vi "DisplayPanel.vi"() -> ()   [LabVIEW 2015]
uses:
  MvLVLib/VIs/CreateU3VHandle.vi
  MvLVLib/VIs/CreateGigEHandle.vi
  MvLVLib/MvCameraControl.lvlib
panel:
  out "Image":T1(plugin-control)
  out "U3VDeviceArray":T2(array[cluster])
  out "GigEDeviceArray":T3(array[cluster])
  in  "pConvertInfo In":T4
  out "PixelFormat":u32
  out "handle out":u64
  in  "handle":u64
  out "PayloadSize":u32
  out "pFrameInfoEx out":T5
  out "nHeight":u32
  out "nWidth":u32
  out "Acquisision Flag":bool
  in  "Trigger Mode":bool
  in  "Continuous":bool
  out "打开标志":bool
  in  "stop":bool
  in  "Trigger Once":bool
  in  "Stop":bool
  in  "Start":bool
  in  "Open Device":bool
  in  "Close Device":bool
  in  "error in (no error) 2":errorcluster caption="错误输入（无错误）"
  in  "Refresh Devices":bool
  in  "Device List":u16(ring) items=["[U3V] _322_sfs_含    22& MV-CS060-10UC-PRO(L25341278)"]
  # "Initialize"
  # "Acquisition"
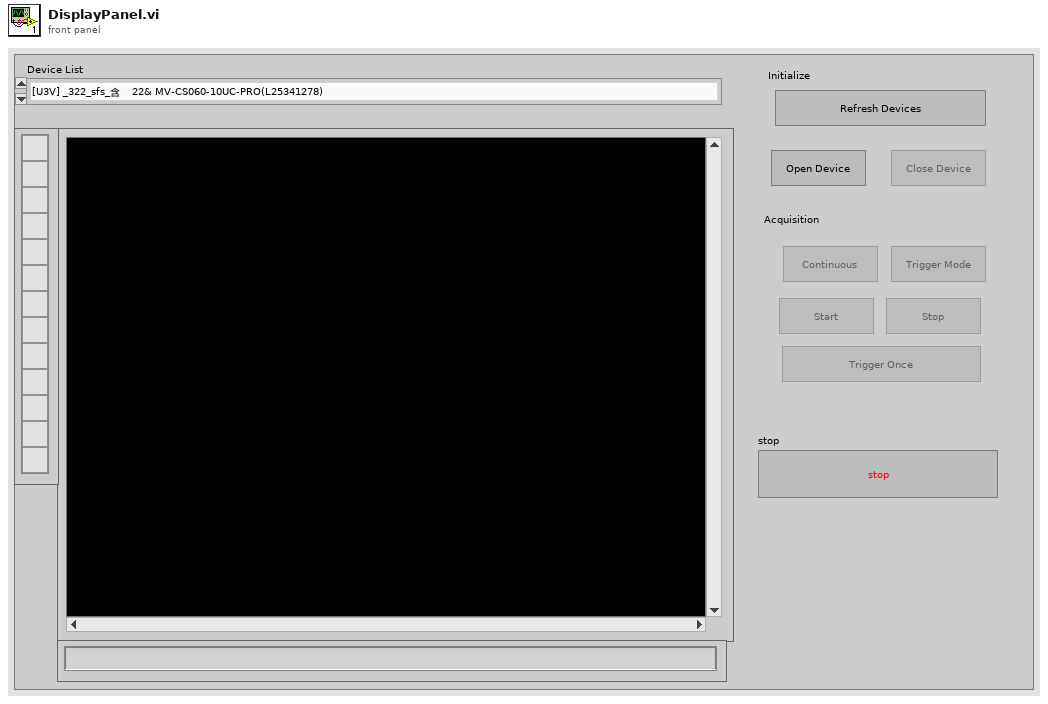
[diagram p1: front panel]
types:
  T1 = typedef "IMAQ Image.ctl" = refnum<image>
  T2 = cluster{"nMajorVer":u16, "nMinorVer":u16, "nMacAddrHigh":u32, "nMacAddrLow":u32, "nTLayerType":u32, "nReserved0":u32, "nReserved1":u32, "nReserved2":u32, "nReserved3":u32, "CrtlInEndPoint":u8, "CrtlOutEndPoint":u8, "StreamEndPoint":u8, "EventEndPoint":u8, "idVendor":u16, "idProduct":u16, "nDeviceNumber":u32, "chDeviceGUID":string, "chVendorName":string, "chModelName":string, "chFamilyName":string, "chDeviceVersion":string, "chManufacturerName":string, "chSerialNumber":string, "chUserDefinedName":string, "nbcdUSB":u32, "nDeviceAddress":u32, "nRes0":u32, "nRes1":u32, "nResAlign":u32}[]
  T3 = cluster{"nMajorVer":u16, "nMinorVer":u16, "nMacAddrHigh":u32, "nMacAddrLow":u32, "nTLayerType":u32, "nReserved0":u32, "nReserved1":u32, "nReserved2":u32, "nReserved3":u32, "nIpCfgOption":u32, "nIpCfgCurrent":u32, "nCurrentIp":u32, "nCurrentSubNetMask":u32, "nDefaultGateWay":u32, "chManualfacturerName":string, "chModelName":string, "chDeviceVersion":string, "chManufacturerSpecificInfo":string, "chSerialNumber":string, "chUserDefinedName":string, "nNetExport":u32, "nRes0":u32, "nRes1":u32, "nRes2":u32, "nRes3":u32}[]
  T4 = cluster{"nWidth":u16, "nHeight":u16, "enSrcPixelType":u32, "nSrcDataLen":u32, "enDstPixelType":u32, "nDstLen":u32, "nDstBufferSize":u32, "nRes0":u32, "nRes1":u32, "nRes2":u32, "nRes3":u32}
  T5 = cluster{"nWidth":u16, "nHeight":u16, "enPixelType":i32, "nFrameNum":u32, "nDevTimeStampHigh":u32, "nDevTimeStampLow":u32, "nReserved0":u32, "nHostTimeStamp":i64, "nFrameLen":u32, "nSecondCount]":u32, "nCycleCount":u32, "nCycleOffset":u32, "fGain":u32, "fExposureTime":u32, "nAverageBrightness":u32, "nRed":u32, "nGreen":u32, "nBlue":u32, "nFrameCounter":u32, "nTriggerIndex":u32, "nInput":u32, "nOutput":u32, "nOffsetX":u32, "nOffsetY":u32, "nReserved[0]":u32, "nReserved[1]":u32, "nReserved[2]":u32, "nReserved[3]":u32, "nReserved[4]":u32, "nReserved[5]":u32, "nReserved[6]":u32, "nReserved[7]":u32, "nReserved[8]":u32, "nReserved[9]":u32, "nReserved[10]":u32, "nReserved[11]":u32, "nReserved[12]":u32, "nReserved[13]":u32, "nReserved[14] 10":u32, "nReserved[15] 11":u32, "nReserved[16] 12":u32, "nReserved[17] 13":u32, "nReserved[18] 14":u32, "nReserved[19] 15":u32, "nReserved[20] 16":u32, "nReserved[21] 17":u32, "nReserved[22] 18":u32, "nReserved[23] 19":u32, "nReserved[24] 20":u32, "nReserved[25] 21":u32, "nReserved[26] 22":u32, "nReserved[27] 23":u32, "nReserved[28] 24":u32, "nReserved[29] 25":u32, "nReserved[30] 26":u32, "nReserved[31] 27":u32, "nReserved[32] 28":u32, "nReserved[33] 29":u32, "nReserved[34] 30":u32, "nReserved[35] 31":u32, "nReserved[36] 32":u32, "nReserved[37] 33":u32, "nReserved[38] 34":u32, "nReserved[39] 35":u32, "nReserved[40] 36":u32}
  T6 = enum8{"Enabled", "Disabled", "Disabled and Grayed Out"}
  T7 = cluster{"nCurValue":u32, "nMax":u32, "nMin":u32, "nInc":u32, "nReserved[0]":u32, "nReserved[1]":u32, "nReserved[2]":u32, "nReserved[3]":u32}
  T8 = cluster{"nCurValue":u32, "nSupportedNum":u32, "nSupportValue[0]":u32, "nSupportValue[1]":u32, "nSupportValue[2]":u32, "nSupportValue[3]":u32, "nSupportValue[4]":u32, "nSupportValue[5]":u32, "nSupportValue[6]":u32, "nSupportValue[7]":u32, "nSupportValue[8]":u32, "nSupportValue[9]":u32, "nSupportValue[10]":u32, "nSupportValue[11]":u32, "nSupportValue[12]":u32, "nSupportValue[13]":u32, "nSupportValue[14]":u32, "nSupportValue[15]":u32, "nSupportValue[16]":u32, "nSupportValue[17]":u32, "nSupportValue[18]":u32, "nSupportValue[19]":u32, "nSupportValue[20]":u32, "nSupportValue[21]":u32, "nSupportValue[22]":u32, "nSupportValue[23]":u32, "nSupportValue[24]":u32, "nSupportValue[25]":u32, "nSupportValue[26]":u32, "nSupportValue[27]":u32, "nSupportValue[28]":u32, "nSupportValue[29]":u32, "nSupportValue[30]":u32, "nSupportValue[31]":u32, "nSupportValue[32]":u32, "nSupportValue[33]":u32, "nSupportValue[34]":u32, "nSupportValue[35]":u32, "nSupportValue[36]":u32, "nSupportValue[37]":u32, "nSupportValue[38]":u32, "nSupportValue[39]":u32, "nSupportValue[40]":u32, "nSupportValue[41]":u32, "nSupportValue[42]":u32, "nSupportValue[43]":u32, "nSupportValue[44]":u32, "nSupportValue[45]":u32, "nSupportValue[46]":u32, "nSupportValue[47]":u32, "nSupportValue[48]":u32, "nSupportValue[49]":u32, "nSupportValue[50]":u32, "nSupportValue[51]":u32, "nSupportValue[52]":u32, "nSupportValue[53]":u32, "nSupportValue[54]":u32, "nSupportValue[55]":u32, "nSupportValue[56]":u32, "nSupportValue[57]":u32, "nSupportValue[58]":u32, "nSupportValue[59]":u32, "nSupportValue[60]":u32, "nSupportValue[61]":u32, "nSupportValue[62]":u32, "nSupportValue[63]":u32, "nReserved[0]":u32, "nReserved[1]":u32, "nReserved[2]":u32, "nReserved[3]":u32}
  T9 = typedef "Image Type" = u32
  T10 = cluster{"nMajorVer":u16, "nMinorVer":u16, "nMacAddrHigh":u32, "nMacAddrLow":u32, "nTLayerType":u32, "nReserved0":u32, "nReserved1":u32, "nReserved2":u32, "nReserved3":u32, "CrtlInEndPoint":u8, "CrtlOutEndPoint":u8, "StreamEndPoint":u8, "EventEndPoint":u8, "idVendor":u16, "idProduct":u16, "nDeviceNumber":u32, "chDeviceGUID":string, "chVendorName":string, "chModelName":string, "chFamilyName":string, "chDeviceVersion":string, "chManufacturerName":string, "chSerialNumber":string, "chUserDefinedName":string, "nbcdUSB":u32, "nDeviceAddress":u32, "nRes0":u32, "nRes1":u32, "nResAlign":u32}
  T11 = cluster{"nMajorVer":u16, "nMinorVer":u16, "nMacAddrHigh":u32, "nMacAddrLow":u32, "nTLayerType":u32, "nReserved0":u32, "nReserved1":u32, "nReserved2":u32, "nReserved3":u32, "nIpCfgOption":u32, "nIpCfgCurrent":u32, "nCurrentIp":u32, "nCurrentSubNetMask":u32, "nDefaultGateWay":u32, "chManualfacturerName":string, "chModelName":string, "chDeviceVersion":string, "chManufacturerSpecificInfo":string, "chSerialNumber":string, "chUserDefinedName":string, "nNetExport":u32, "nRes0":u32, "nRes1":u32, "nRes2":u32, "nRes3":u32}
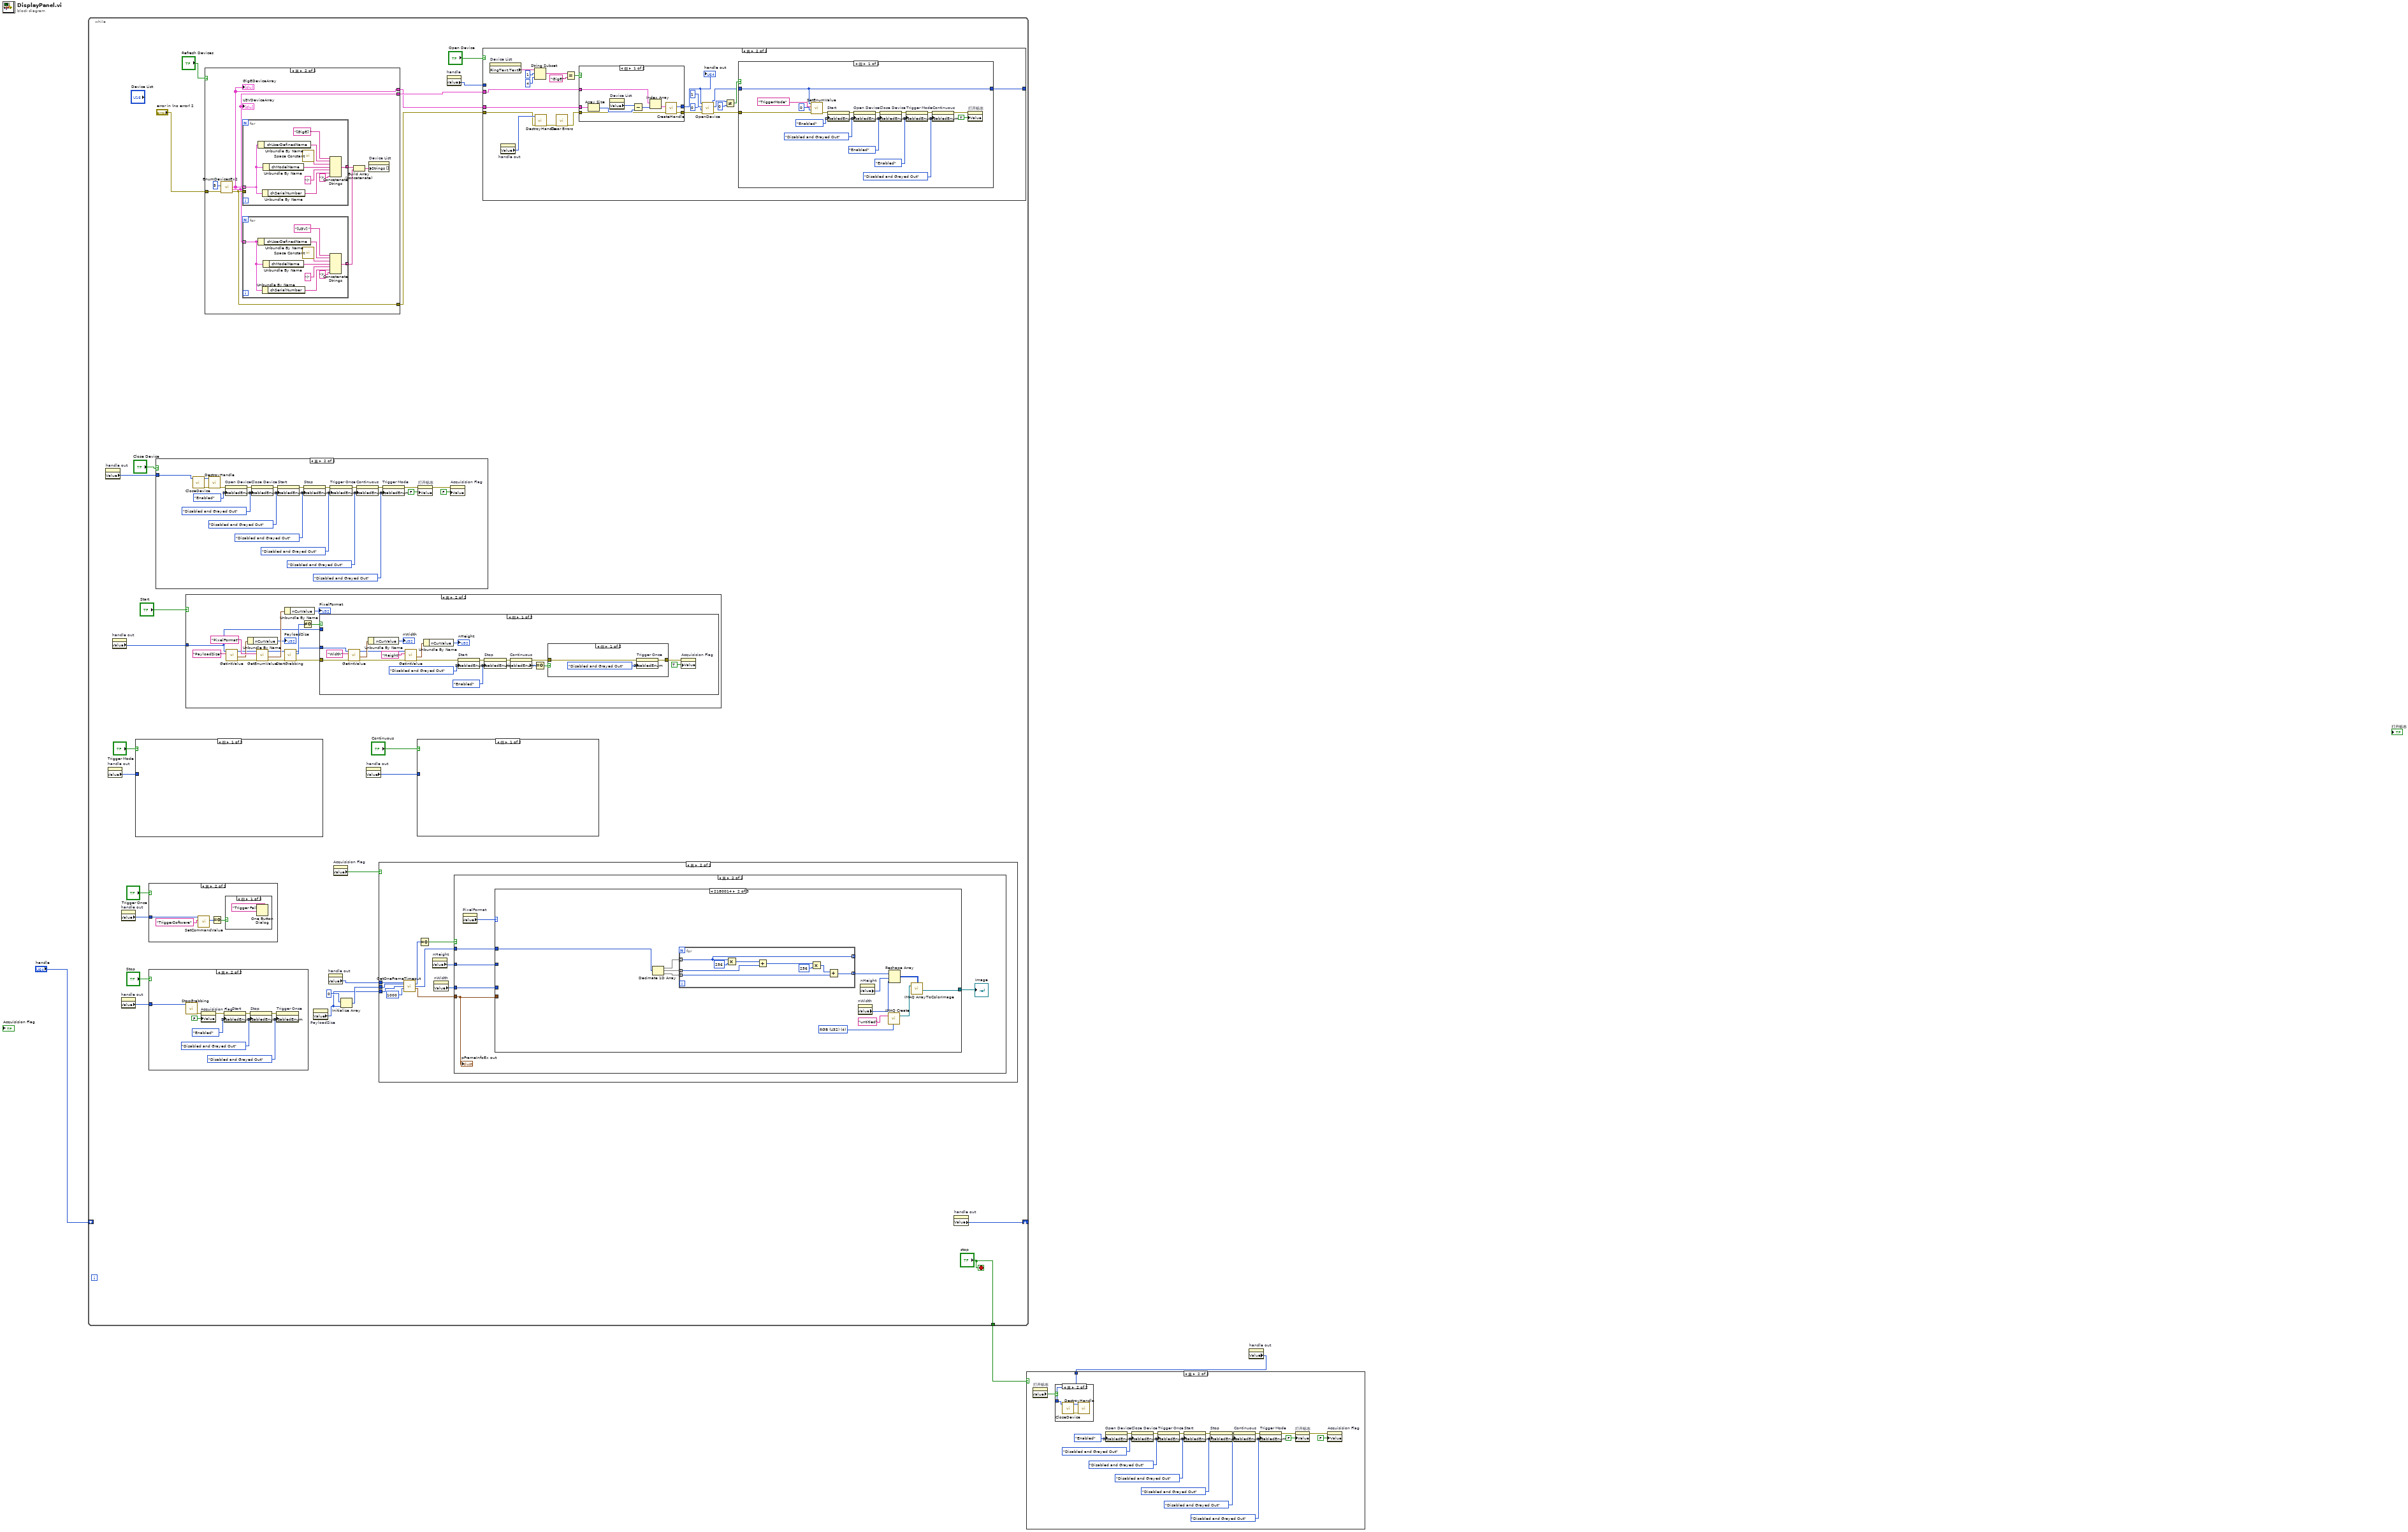
[diagram p0: block diagram]
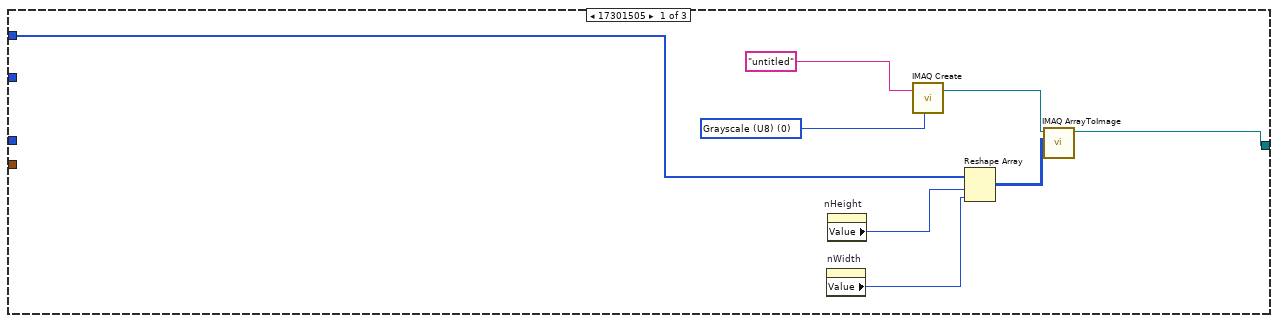
[diagram p6: hidden frame]
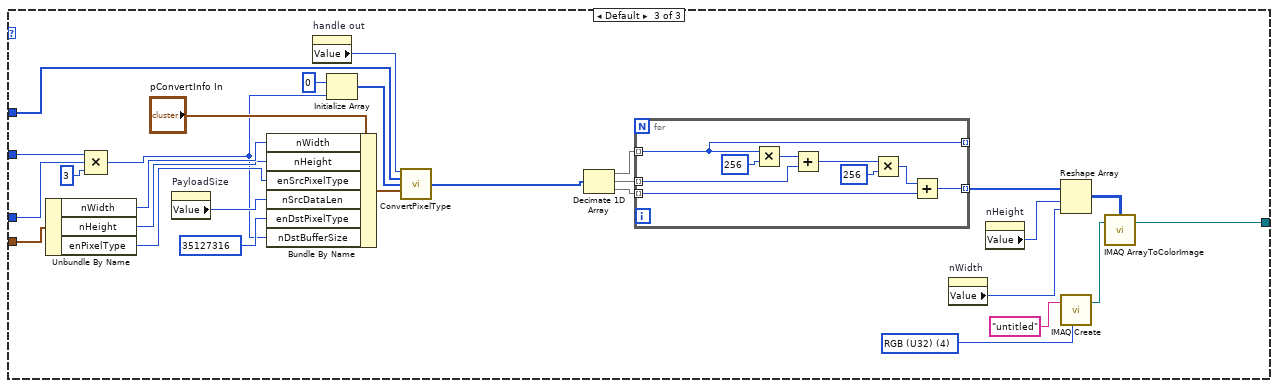
[diagram p7: hidden frame]
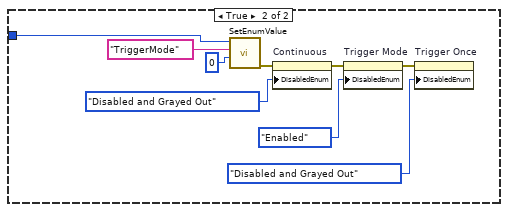
[diagram p9: hidden frame]
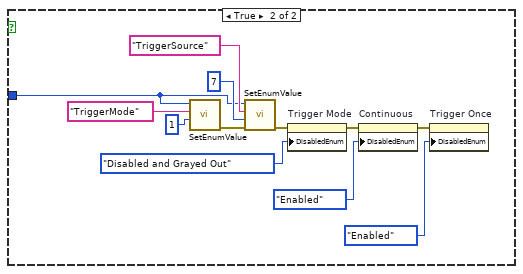
[diagram p10: hidden frame]
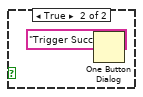
[diagram p12: hidden frame]
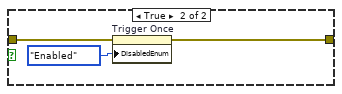
[diagram p14: hidden frame]
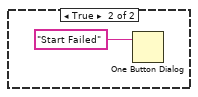
[diagram p15: hidden frame]
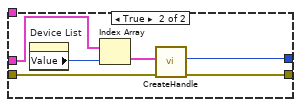
[diagram p18: hidden frame]
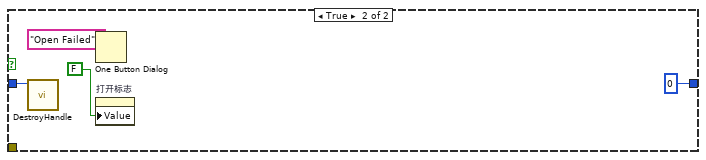
[diagram p19: hidden frame]
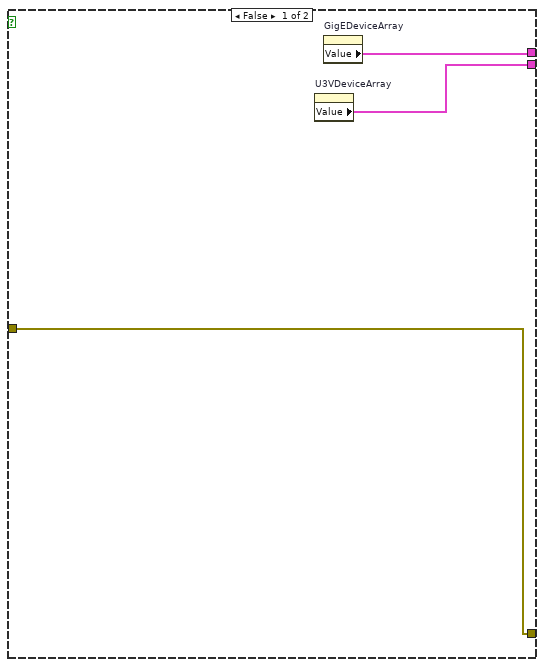
[diagram p20: hidden frame]
diagram:
  n1 = while {
    tunnel: ["stop"] -> w3
    shift-right: [w17] -> _
    shift-left: "handle" -> [_]
    stop <- "stop" stop-if-true
    n2 = property on="handle out" class="DigNum (严格)"() -> ("Value"=w15:u64)  [unwired: 2 in, 2 out]
    n3 = property on="handle out" class="DigNum (严格)"() -> ("Value"=w10:u64)  [unwired: 2 in, 2 out]
    n4 = property on="handle out" class="DigNum (严格)"() -> ("Value"=w11:u64)  [unwired: 2 in, 2 out]
    n5 = property on="handle out" class="DigNum (严格)"() -> ("Value"=w14:u64)  [unwired: 2 in, 2 out]
    n6 = property on="handle out" class="DigNum (严格)"() -> ("Value"=w13:u64)  [unwired: 2 in, 2 out]
    n7 = case shown="假" "Trigger Mode" {
      tunnel: w10 -> [_ w130]
      frame False {
      }
      frame True {
        n8 = call "SetEnumValue.vi"("nValue"=u32 1, "strKey"="TriggerMode", "handle"=w130) -> ("error out"=w136:errorcluster)  [unwired: 6 in, 2 out]
        n9 = call "SetEnumValue.vi"("error in (no error)"=w136, "nValue"=u32 7, "strKey"="TriggerSource", "handle"=w130) -> ("error out"=w135:errorcluster)  [unwired: 5 in, 2 out]
        n10 = property on="Trigger Mode" class="Bool"(error in=w135, "DisabledEnum"=T6."Disabled and Grayed Out" ("禁用")) -> (error out=w134:errorcluster)  [unwired: 1 in, 1 out]
        n11 = property on="Continuous" class="Bool"(error in=w134, "DisabledEnum"=T6."Enabled" ("禁用")) -> (error out=w132:errorcluster)  [unwired: 1 in, 1 out]
        n12 = property on="Trigger Once" class="Bool"(error in=w132, "DisabledEnum"=T6."Enabled" ("禁用")) -> ()  [unwired: 1 in, 2 out]
      }
    }
    n13 = case shown="真" "Trigger Once" {
      tunnel: w14 -> [_ w145]
      frame False {
      }
      frame True {
        n14 = call "SetCommandValue.vi"("strValue"="TriggerSoftware", "handle"=w145) -> ("function return"=w143:i32)  [unwired: 7 in, 2 out]
        n15 = Equal To 0?(x=w143) -> (x = 0?=w142:bool)
        n16 = case shown="假" w142 {
          frame False {
            n17 = One Button Dialog(message="Trigger Failed") -> ()  [unwired: 1 in, 1 out]
          }
          frame True {
            n18 = One Button Dialog(message="Trigger Success") -> ()  [unwired: 1 in, 1 out]
          }
        }
      }
    }
    n19 = case shown="真" "Stop" {
      tunnel: w13 -> [_ w120]
      frame False {
      }
      frame True {
        n20 = call "StopGrabbing.vi"("handle"=w120) -> ("error out"=w119:errorcluster)  [unwired: 8 in, 2 out]
        n21 = property on="Acquisision Flag" class="Bool (严格)"(error in=w119, "Value"=FALSE ("采集标志")) -> (error out=w114:errorcluster)  [unwired: 1 in, 1 out]
        n22 = property on="Start" class="Bool"(error in=w114, "DisabledEnum"=T6."Enabled" ("禁用")) -> (error out=w113:errorcluster)  [unwired: 1 in, 1 out]
        n23 = property on="Stop" class="Bool"(error in=w113, "DisabledEnum"=T6."Disabled and Grayed Out" ("禁用")) -> (error out=w112:errorcluster)  [unwired: 1 in, 1 out]
        n24 = property on="Trigger Once" class="Bool"(error in=w112, "DisabledEnum"=T6."Disabled and Grayed Out" ("禁用")) -> ()  [unwired: 1 in, 2 out]
      }
    }
    n25 = case shown="真" "Close Device" {
      tunnel: w15 -> [_ w191]
      frame False {
      }
      frame True {
        n26 = call "CloseDevice.vi"("handle"=w191) -> ("error out"=w193:errorcluster, "handle out"=w190:u64)  [unwired: 8 in, 1 out]
        n27 = call "DestroyHandle.vi"("error in (no error)"=w193, "handle"=w190) -> ("error out"=w192:errorcluster)  [unwired: 8 in, 1 out]
        n28 = property on="Open Device" class="Bool"(error in=w192, "DisabledEnum"=T6."Enabled" ("禁用")) -> (error out=w206:errorcluster)  [unwired: 1 in, 1 out]
        n29 = property on="Close Device" class="Bool"(error in=w206, "DisabledEnum"=T6."Disabled and Grayed Out" ("禁用")) -> (error out=w205:errorcluster)  [unwired: 1 in, 1 out]
        n30 = property on="Start" class="Bool"(error in=w205, "DisabledEnum"=T6."Disabled and Grayed Out" ("禁用")) -> (error out=w204:errorcluster)  [unwired: 1 in, 1 out]
        n31 = property on="Stop" class="Bool"(error in=w204, "DisabledEnum"=T6."Disabled and Grayed Out" ("禁用")) -> (error out=w203:errorcluster)  [unwired: 1 in, 1 out]
        n32 = property on="Trigger Once" class="Bool"(error in=w203, "DisabledEnum"=T6."Disabled and Grayed Out" ("禁用")) -> (error out=w200:errorcluster)  [unwired: 1 in, 1 out]
        n33 = property on="Continuous" class="Bool"(error in=w200, "DisabledEnum"=T6."Disabled and Grayed Out" ("禁用")) -> (error out=w198:errorcluster)  [unwired: 1 in, 1 out]
        n34 = property on="Trigger Mode" class="Bool"(error in=w198, "DisabledEnum"=T6."Disabled and Grayed Out" ("禁用")) -> (error out=w197:errorcluster)  [unwired: 1 in, 1 out]
        n35 = property on="打开标志" class="Bool (严格)"(error in=w197, "Value"=FALSE ("打开标志")) -> (error out=w195:errorcluster)  [unwired: 1 in, 1 out]
        n36 = property on="Acquisision Flag" class="Bool (严格)"(error in=w195, "Value"=FALSE ("采集标志")) -> ()  [unwired: 1 in, 2 out]
      }
    }
    n37 = case shown="真" "Start" {
      tunnel: w11 -> [_ w152]
      frame False {
      }
      frame True {
        n38 = call "GetIntValue.vi"("strKey"="PayloadSize", "handle"=w152) -> ("error out"=w158:errorcluster, "pIntValue out"=w154:T7, "handle out"=w150:u64)  [unwired: 6 in, 1 out]
        n39 = Unbundle By Name(w154) -> ("nCurValue"=→"PayloadSize":u32)
        n40 = call "GetEnumValue.vi"("error in (no error)"=w158, "strKey"="PixelFormat", "handle"=w150) -> ("error out"=w157:errorcluster, "pEnumValue out"=w159:T8, "handle out"=w149:u64)  [unwired: 5 in, 1 out]
        n41 = Unbundle By Name(w159) -> ("nCurValue"=→"PixelFormat":u32)
        n42 = call "StartGrabbing.vi"("error in (no error)"=w157, "handle"=w149) -> ("error out"=w156:errorcluster, "function return"=w162:i32, "handle out"=w148:u64)  [unwired: 7 in]
        n43 = Not Equal To 0?(x=w162) -> (x != 0?=w161:bool)
        n44 = case shown="假" w161 {
          tunnel: w152 -> [_ _]
          tunnel: w156 -> [w165 _]
          tunnel: w148 -> [w164 _]
          frame False {
            n45 = call "GetIntValue.vi"("error in (no error)"=w165, "strKey"="Width", "handle"=w164) -> ("error out"=w172:errorcluster, "pIntValue out"=w166:T7, "handle out"=w163:u64)  [unwired: 5 in, 1 out]
            n46 = Unbundle By Name(w166) -> ("nCurValue"=→"nWidth":u32)
            n47 = call "GetIntValue.vi"("error in (no error)"=w172, "strKey"="Height", "handle"=w163) -> ("error out"=w171:errorcluster, "pIntValue out"=w169:T7)  [unwired: 5 in, 2 out]
            n48 = Unbundle By Name(w169) -> ("nCurValue"=→"nHeight":u32)
            n49 = property on="Start" class="Bool"(error in=w171, "DisabledEnum"=T6."Disabled and Grayed Out" ("禁用")) -> (error out=w181:errorcluster)  [unwired: 1 in, 1 out]
            n50 = property on="Stop" class="Bool"(error in=w181, "DisabledEnum"=T6."Enabled" ("禁用")) -> (error out=w167:errorcluster)  [unwired: 1 in, 1 out]
            n51 = property on="Continuous" class="Bool"(error in=w167) -> (error out=w177:errorcluster, "DisabledEnum"=w178:T6)  [unwired: 1 in, 1 out]
            n52 = Equal To 0?(x=w178) -> (x = 0?=w179:bool)
            n53 = case shown="假" w179 {
              tunnel: w177 -> [w184 w187]
              tunnel: [w183 w186] -> w176
              frame False {
                n54 = property on="Trigger Once" class="Bool"(error in=w184, "DisabledEnum"=T6."Disabled and Grayed Out" ("禁用")) -> (error out=w183:errorcluster)  [unwired: 1 in, 1 out]
              }
              frame True {
                n55 = property on="Trigger Once" class="Bool"(error in=w187, "DisabledEnum"=T6."Enabled" ("禁用")) -> (error out=w186:errorcluster)  [unwired: 1 in, 1 out]
              }
            }
            n56 = property on="Acquisision Flag" class="Bool (严格)"(error in=w176, "Value"=TRUE ("采集标志")) -> ()  [unwired: 1 in, 2 out]
          }
          frame True {
            n57 = One Button Dialog(message="Start Failed") -> ()  [unwired: 1 in, 1 out]
          }
        }
      }
    }
    n58 = case shown="真" "Refresh Devices" {
      tunnel: [w271 w279] -> w19
      tunnel: "error in (no error) 2" -> [w271 w278]
      tunnel: [w269 w273] -> w5
      tunnel: [w270 w274] -> w4
      frame False {
        n59 = property on="U3VDeviceArray" class="Arr (严格)"() -> ("Value"=w269:T2)  [unwired: 2 in, 2 out]
        n60 = property on="GigEDeviceArray" class="Arr (严格)"() -> ("Value"=w270:T3)  [unwired: 2 in, 2 out]
      }
      frame True {
        n61 = call "EnumDevicesEx2.vi"("nLayerType"=5, "error in (no error)"=w278) -> ("GigEDeviceArray"=w274:T3, "U3VDeviceArray"=w273:T2, "error out"=w279:errorcluster)  [unwired: 9 in, 2 out]
        "GigEDeviceArray" <- w274
        "U3VDeviceArray" <- w273
        n62 = for {
          tunnel: w279 -> [_]
          tunnel: w274 -> [w291] mode=indexing
          tunnel: [w290] -> w277 mode=indexing
          n63 = Unbundle By Name(w291) -> ("chUserDefinedName"=w294:string)
          n64 = Unbundle By Name(w291) -> ("chSerialNumber"=w292:string)
          n65 = Unbundle By Name(w291) -> ("chModelName"=w293:string)
          n66 = call <vilib>:"Space Constant.vi"() -> ("String"=w297:string)
          n67 = Concatenate Strings("[GigE] " ("字符串"), w294, w297, w293, "(" ("字符串"), w292, ")" ("字符串")) -> (w290:string)
        }
        n68 = for {
          tunnel: w273 -> [w284] mode=indexing
          tunnel: [w281] -> w276 mode=indexing
          n69 = Unbundle By Name(w284) -> ("chUserDefinedName"=w288:string)
          n70 = Unbundle By Name(w284) -> ("chSerialNumber"=w283:string)
          n71 = Unbundle By Name(w284) -> ("chModelName"=w286:string)
          n72 = call <vilib>:"Space Constant.vi"() -> ("String"=w287:string)
          n73 = Concatenate Strings("[U3V] " ("字符串"), w288, w287, w286, "(" ("字符串"), w283, ")" ("字符串")) -> (w281:string)
        }
        n74 = Build Array (concatenate)(w277, w276) -> (w275:string[])
        n75 = property on="Device List" class="Ring (严格)"("Strings []"=w275) -> ()  [unwired: 2 in, 2 out]
      }
    }
    n76 = property on="PayloadSize" class="DigNum (严格)"() -> ("Value"=w6:u32)  [unwired: 2 in, 2 out]
    n77 = property on="handle out" class="DigNum (严格)"() -> ("Value"=w12:u64)  [unwired: 2 in, 2 out]
    n78 = property on="Acquisision Flag" class="Bool (严格)"() -> ("Value"=w21:bool)  [unwired: 2 in, 2 out]
    n79 = Initialize Array(u8 0 ("元素"), w6) -> (w7:u8[])
    n80 = property on="handle out" class="DigNum (严格)"() -> ("Value"=w9:u64)  [unwired: 2 in, 2 out]
    n81 = case shown="真" w21 {
      tunnel: w12 -> [_ w35]
      tunnel: w7 -> [_ w34]
      tunnel: w6 -> [_ w33]
      frame False {
      }
      frame True {
        n82 = call "GetOneFrameTimeout.vi"("handle"=w35, "pData"=w34, "nDataSize"=w33, "nMsec"=1000) -> ("function return"=w32:i32, "pData Out"=w31:u8[], "pFrameInfoEx out"=w30:T5)  [unwired: 7 in, 2 out]
        n83 = Equal To 0?(x=w32) -> (x = 0?=w39:bool)
        n84 = property on="nHeight" class="DigNum (严格)"() -> ("Value"=w37:u32)  [unwired: 2 in, 2 out]
        n85 = property on="nWidth" class="DigNum (严格)"() -> ("Value"=w38:u32)  [unwired: 2 in, 2 out]
        n86 = case shown="真" w39 {
          tunnel: w31 -> [_ w45]
          tunnel: w38 -> [_ w43]
          tunnel: w37 -> [_ w44]
          tunnel: w30 -> [_ w41]
          frame False {
          }
          frame True {
            n87 = property on="PixelFormat" class="DigNum (严格)"() -> ("Value"=w42:u32)  [unwired: 2 in, 2 out]
            n88 = case shown="2180014" w42 {
              tunnel: w45 -> [w46 w57 w99]
              tunnel: w44 -> [_ _ w96]
              tunnel: w43 -> [_ _ w95]
              tunnel: w41 -> [_ _ w87]
              tunnel: [w47 w56 w75] -> w40
              frame 17301505 {
                w53 = T9 0 items=["Grayscale (U8)", "Grayscale (I16)", "Grayscale (SGL)", "Complex (CSG)", "RGB (U32)", "HSL (U32)", "RGB (U64)", "Grayscale (U16)"] ("Image Type")
                n89 = property on="nWidth" class="DigNum (严格)"() -> ("Value"=w48:u32)  [unwired: 2 in, 2 out]
                n90 = property on="nHeight" class="DigNum (严格)"() -> ("Value"=w49:u32)  [unwired: 2 in, 2 out]
                n91 = call "IMAQ Create"("Image Name"="untitled", "Image Type"=w53) -> ("New Image"=w51:T1)  [unwired: 3 in, 1 out]
                n92 = Reshape Array(w46, w49, w48) -> (w50:u8[][])
                n93 = call "IMAQ ArrayToImage"("Image Pixels (U8)"=w50, "Image"=w51) -> ("Image Out"=w47:T1)  [unwired: 8 in, 1 out]
              }
              frame 35127316 {
                w65 = T9 4 items=["Grayscale (U8)", "Grayscale (I16)", "Grayscale (SGL)", "Complex (CSG)", "RGB (U32)", "HSL (U32)", "RGB (U64)", "Grayscale (U16)"] ("Image Type")
                n94 = Decimate 1D Array(w57) -> (w58:u8[], w59:u8[], w60:u8[])
                n95 = for {
                  tunnel: w58 -> [w66] mode=indexing
                  tunnel: w59 -> [w72] mode=indexing
                  tunnel: w60 -> [w68] mode=indexing
                  tunnel: [w67] -> w61 mode=indexing
                  tunnel: [w66] -> _ mode=indexing
                  n96 = Multiply(x=w66, y=256) -> (x*y=w73:i32)
                  n97 = Add(x=w73, y=w72) -> (x+y=w71:i32)
                  n98 = Multiply(x=w71, y=256) -> (x*y=w69:i32)
                  n99 = Add(x=w69, y=w68) -> (x+y=w67:i32)
                }
                n100 = property on="nWidth" class="DigNum (严格)"() -> ("Value"=w54:u32)  [unwired: 2 in, 2 out]
                n101 = property on="nHeight" class="DigNum (严格)"() -> ("Value"=w55:u32)  [unwired: 2 in, 2 out]
                n102 = call "IMAQ Create"("Image Name"="untitled", "Image Type"=w65) -> ("New Image"=w63:T1)  [unwired: 3 in, 1 out]
                n103 = Reshape Array(w61, w55, w54) -> (w62:i32[][])
                n104 = call "IMAQ ArrayToColorImage"("Image Pixels (U32)"=w62, "Image"=w63) -> ("Image Out"=w56:T1)  [unwired: 3 in, 1 out]
              }
              frame Default {
                w86 = T9 4 items=["Grayscale (U8)", "Grayscale (I16)", "Grayscale (SGL)", "Complex (CSG)", "RGB (U32)", "HSL (U32)", "RGB (U64)", "Grayscale (U16)"] ("Image Type")
                n105 = Unbundle By Name(w87) -> ("nWidth"=w94:u16, "nHeight"=w93:u16, "enPixelType"=w92:i32)
                n106 = Compound Arithmetic op=MULTIPLY(w96, w95, u32 3 ("值")) -> (w89:u32)
                n107 = property on="PayloadSize" class="DigNum (严格)"() -> ("Value"=w91:u32)  [unwired: 2 in, 2 out]
                n108 = Bundle By Name(cluster="pConvertInfo In", "nWidth"=w94, "nHeight"=w93, "enSrcPixelType"=w92, "nSrcDataLen"=w91, "enDstPixelType"=u32 35127316, "nDstBufferSize"=w89) -> (w88:T4)
                n109 = property on="handle out" class="DigNum (严格)"() -> ("Value"=w100:u64)  [unwired: 2 in, 2 out]
                n110 = Initialize Array(u8 0 ("元素"), w89) -> (w98:u8[])
                n111 = call "ConvertPixelType.vi"("handle"=w100, "pSrcData"=w99, "pDstBuf In"=w98, "pConvertInfo In"=w88) -> ("pDstBuf Out"=w78:u8[])  [unwired: 7 in, 4 out]
                n112 = Decimate 1D Array(w78) -> (w79:u8[], w80:u8[], w81:u8[])
                n113 = for {
                  tunnel: w79 -> [w103] mode=indexing
                  tunnel: w80 -> [w109] mode=indexing
                  tunnel: w81 -> [w105] mode=indexing
                  tunnel: [w104] -> w82 mode=indexing
                  tunnel: [w103] -> _ mode=indexing
                  n114 = Multiply(x=w103, y=256) -> (x*y=w110:i32)
                  n115 = Add(x=w110, y=w109) -> (x+y=w108:i32)
                  n116 = Multiply(x=w108, y=256) -> (x*y=w106:i32)
                  n117 = Add(x=w106, y=w105) -> (x+y=w104:i32)
                }
                n118 = property on="nWidth" class="DigNum (严格)"() -> ("Value"=w76:u32)  [unwired: 2 in, 2 out]
                n119 = property on="nHeight" class="DigNum (严格)"() -> ("Value"=w77:u32)  [unwired: 2 in, 2 out]
                n120 = Reshape Array(w82, w77, w76) -> (w83:i32[][])
                n121 = call "IMAQ Create"("Image Name"="untitled", "Image Type"=w86) -> ("New Image"=w84:T1)  [unwired: 3 in, 1 out]
                n122 = call "IMAQ ArrayToColorImage"("Image Pixels (U32)"=w83, "Image"=w84) -> ("Image Out"=w75:T1)  [unwired: 3 in, 1 out]
              }
            }
            "Image" <- w40
            "pFrameInfoEx out" <- w41
          }
        }
      }
    }
    n123 = case shown="假" "Continuous" {
      tunnel: w9 -> [_ w121]
      frame False {
      }
      frame True {
        n124 = call "SetEnumValue.vi"("nValue"=u32 0, "strKey"="TriggerMode", "handle"=w121) -> ("error out"=w122:errorcluster)  [unwired: 6 in, 2 out]
        n125 = property on="Continuous" class="Bool"(error in=w122, "DisabledEnum"=T6."Disabled and Grayed Out" ("禁用")) -> (error out=w126:errorcluster)  [unwired: 1 in, 1 out]
        n126 = property on="Trigger Mode" class="Bool"(error in=w126, "DisabledEnum"=T6."Enabled" ("禁用")) -> (error out=w124:errorcluster)  [unwired: 1 in, 1 out]
        n127 = property on="Trigger Once" class="Bool"(error in=w124, "DisabledEnum"=T6."Disabled and Grayed Out" ("禁用")) -> ()  [unwired: 1 in, 2 out]
      }
    }
    n128 = property on="handle" class="DigNum (严格)"() -> ("Value"=w16:u64)  [unwired: 2 in, 2 out]
    n129 = case shown="真" "Open Device" {
      tunnel: [w211 w226] -> _
      tunnel: w16 -> [w211 _]
      tunnel: w19 -> [_ w214]
      tunnel: w5 -> [_ w217]
      tunnel: w4 -> [_ w216]
      frame False {
      }
      frame True {
        n130 = property on="Device List" class="Ring (严格)"() -> ("RingText.Text"=w225:string)  [unwired: 2 in, 2 out]
        n131 = property on="handle out" class="DigNum (严格)"() -> ("Value"=w215:u64)  [unwired: 2 in, 2 out]
        n132 = String Subset(string=w225, offset (0)=1 ("偏移量(0)"), length (rest)=4 ("长度（剩余）")) -> (substring=w222:string)
        n133 = call "DestroyHandle.vi"("error in (no error)"=w214, "handle"=w215) -> ("error out"=w213:errorcluster)  [unwired: 8 in, 1 out]
        n134 = call <vilib>:"Clear Errors.vi"("error in (no error)"=w213) -> ("error out"=w212:errorcluster)  [unwired: 5 in, 1 out]
        n135 = Equal?(x=w222, y="GigE") -> (x = y?=w221:bool)
        n136 = case shown="假" w221 {
          tunnel: [w236 w245] -> w231
          tunnel: [w235 w244] -> w227
          tunnel: w216 -> [w240 w247]
          tunnel: w212 -> [w237 w246]
          tunnel: w217 -> [w242 _]
          frame False {
            n137 = Array Size(array=w240) -> (size(s)=w239:i32)
            n138 = property on="Device List" class="Ring (严格)"() -> ("Value"=w241:u16)  [unwired: 2 in, 2 out]
            n139 = Subtract(x=w241, y=w239) -> (x-y=w238:i32)
            n140 = Index Array(array=w242, index=w238) -> (element=w234:T10)
            n141 = call-poly "CreateHandle.vi"("error in (no error)"=w237, "U3VDevice"=w234) -> ("error out"=w236:errorcluster, "handle"=w235:u64)  [unwired: 6 in, 1 out]
          }
          frame True {
            n142 = property on="Device List" class="Ring (严格)"() -> ("Value"=w248:u16)  [unwired: 2 in, 2 out]
            n143 = Index Array(array=w247, index=w248) -> (element=w243:T11)
            n144 = call-poly "CreateHandle.vi"("error in (no error)"=w246, "GigEDevice"=w243) -> ("error out"=w245:errorcluster, "handle"=w244:u64)  [unwired: 6 in, 1 out]
          }
        }
        "handle out" <- w227
        n145 = call "OpenDevice.vi"("error in (no error)"=w231, "nSwitchoverKey"=u16 0, "nAccessMode"=u32 1, "handle"=w227) -> ("error out"=w228:errorcluster, "return"=w219:i32, "handle out"=w218:u64)  [unwired: 5 in]
        n146 = Not Equal?(x=w219, y=0) -> (x != y?=w232:bool)
        n147 = case shown="假" w232 {
          tunnel: w218 -> [w249 w266]
          tunnel: w228 -> [w250 _]
          tunnel: [w249 u64 0 ("handle")] -> w226
          frame False {
            n148 = call "SetEnumValue.vi"("error in (no error)"=w250, "nValue"=u32 0, "strKey"="TriggerMode", "handle"=w249) -> ("error out"=w261:errorcluster)  [unwired: 5 in, 2 out]
            n149 = property on="Start" class="Bool"(error in=w261, "DisabledEnum"=T6."Enabled" ("禁用")) -> (error out=w259:errorcluster)  [unwired: 1 in, 1 out]
            n150 = property on="Open Device" class="Bool"(error in=w259, "DisabledEnum"=T6."Disabled and Grayed Out" ("禁用")) -> (error out=w258:errorcluster)  [unwired: 1 in, 1 out]
            n151 = property on="Close Device" class="Bool"(error in=w258, "DisabledEnum"=T6."Enabled" ("禁用")) -> (error out=w255:errorcluster)  [unwired: 1 in, 1 out]
            n152 = property on="Trigger Mode" class="Bool"(error in=w255, "DisabledEnum"=T6."Enabled" ("禁用")) -> (error out=w253:errorcluster)  [unwired: 1 in, 1 out]
            n153 = property on="Continuous" class="Bool"(error in=w253, "DisabledEnum"=T6."Disabled and Grayed Out" ("禁用")) -> (error out=w251:errorcluster)  [unwired: 1 in, 1 out]
            n154 = property on="打开标志" class="Bool (严格)"(error in=w251, "Value"=TRUE ("布尔")) -> ()  [unwired: 1 in, 2 out]
          }
          frame True {
            n155 = call "DestroyHandle.vi"("handle"=w266) -> ()  [unwired: 9 in, 2 out]
            n156 = One Button Dialog(message="Open Failed") -> ()  [unwired: 1 in, 1 out]
            n157 = property on="打开标志" class="Bool (严格)"("Value"=FALSE) -> ()  [unwired: 2 in, 2 out]
          }
        }
      }
    }
    n158 = property on="handle out" class="DigNum (严格)"() -> ("Value"=w17:u64)  [unwired: 2 in, 2 out]
  }
  n159 = property on="handle out" class="DigNum (严格)"() -> ("Value"=w1:u64)  [unwired: 2 in, 2 out]
  n160 = case shown="真" w3 {
    tunnel: w1 -> [_ w311]
    frame False {
    }
    frame True {
      n161 = property on="打开标志" class="Bool (严格)"() -> ("Value"=w302:bool)  [unwired: 2 in, 2 out]
      n162 = case shown="真" w302 {
        tunnel: w311 -> [_ w318]
        frame False {
        }
        frame True {
          n163 = call "CloseDevice.vi"("handle"=w318) -> ("error out"=w319:errorcluster, "handle out"=w317:u64)  [unwired: 8 in, 1 out]
          n164 = call "DestroyHandle.vi"("error in (no error)"=w319, "handle"=w317) -> ()  [unwired: 8 in, 2 out]
        }
      }
      n165 = property on="Open Device" class="Bool"("DisabledEnum"=T6."Enabled" ("禁用")) -> (error out=w310:errorcluster)  [unwired: 2 in, 1 out]
      n166 = property on="Close Device" class="Bool"(error in=w310, "DisabledEnum"=T6."Disabled and Grayed Out" ("禁用")) -> (error out=w309:errorcluster)  [unwired: 1 in, 1 out]
      n167 = property on="Trigger Once" class="Bool"(error in=w309, "DisabledEnum"=T6."Disabled and Grayed Out" ("禁用")) -> (error out=w308:errorcluster)  [unwired: 1 in, 1 out]
      n168 = property on="Start" class="Bool"(error in=w308, "DisabledEnum"=T6."Disabled and Grayed Out" ("禁用")) -> (error out=w307:errorcluster)  [unwired: 1 in, 1 out]
      n169 = property on="Stop" class="Bool"(error in=w307, "DisabledEnum"=T6."Disabled and Grayed Out" ("禁用")) -> (error out=w306:errorcluster)  [unwired: 1 in, 1 out]
      n170 = property on="Continuous" class="Bool"(error in=w306, "DisabledEnum"=T6."Disabled and Grayed Out" ("禁用")) -> (error out=w304:errorcluster)  [unwired: 1 in, 1 out]
      n171 = property on="Trigger Mode" class="Bool"(error in=w304, "DisabledEnum"=T6."Disabled and Grayed Out" ("禁用")) -> (error out=w299:errorcluster)  [unwired: 1 in, 1 out]
      n172 = property on="打开标志" class="Bool (严格)"(error in=w299, "Value"=FALSE ("打开标志")) -> (error out=w298:errorcluster)  [unwired: 1 in, 1 out]
      n173 = property on="Acquisision Flag" class="Bool (严格)"(error in=w298, "Value"=FALSE ("采集标志")) -> ()  [unwired: 1 in, 2 out]
    }
  }
